vi "Zeile faerben.vi"(8 "error in (no error)":errorcluster caption="Fehler (Eingang, kein Fehler)", 9 "Offset für Start":i32, 10 "Anzahl":i32, 11 "Table (Eingang)":refnum<vi>) -> (0 "error out":errorcluster caption="Fehler (Ausgang)")   [LabVIEW 2020, in "FT-IR.lvlib" / "Spanfaktor.lvlib"]
uses:
  Spanfaktor.lvlib
  <vilib>/Utility/miscctls.llb/LVRowAndColumnTypeDef.ctl
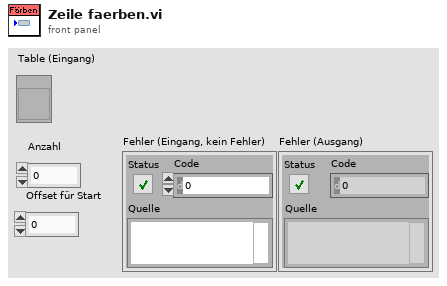
[diagram p1: front panel]
types:
  T1 = typedef "LVRowAndColumnTypeDef.ctl" = cluster{"Row":i32, "Column":i32}
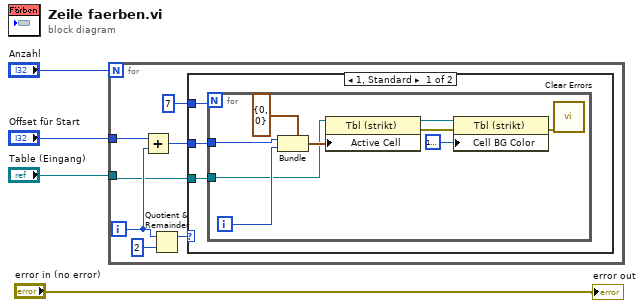
[diagram p0: block diagram]
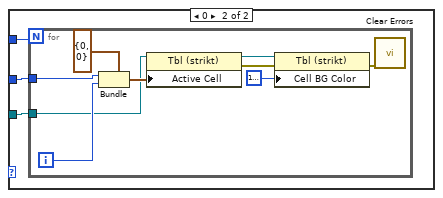
[diagram p2: hidden frame]
diagram:
  n1 = for {
    N: "Anzahl" -> [_]
    tunnel: "Table (Eingang)" -> [w8]
    tunnel: "Offset für Start" -> [w5]
    i -> [w9]
    n2 = Add(x=w5, y=w9) -> (x+y=w6:i32)
    n3 = Quotient & Remainder(x=w9, y=2) -> (x-y*floor(x/y)=w10:i32)  [unwired: 1 out]
    n4 = case shown="1, Standard" w10 {
      tunnel: w8 -> [w14 w26]
      tunnel: w6 -> [w13 w25]
      tunnel: 7 -> [w12 w24]
      frame 1, Default {
        n5 = for {
          N: w12 -> [_]
          tunnel: w14 -> [w18]
          tunnel: w13 -> [w20]
          i -> [w19]
          n6 = Bundle(cluster=T1 {"Row"=0, "Column"=0} ("Aktive Zelle:Aktive Zelle"), "Row"=w20, "Column"=w19) -> (w21:T1)
          n7 = property class="Tbl (strikt)"(reference=w18, "Active Cell"=w21) -> (reference out=w17:refnum<vi>, error out=w15:errorcluster)  [unwired: 1 in]
          n8 = property class="Tbl (strikt)"(reference=w17, error in=w15, "Cell BG Color"=u32 16777225) -> (error out=w16:errorcluster)  [unwired: 1 out]
          n9 = call <vilib>:"Clear Errors.vi"("error in (no error)"=w16) -> ()  [unwired: 5 in, 2 out]
        }
      }
      frame 0 {
        n10 = for {
          N: w24 -> [_]
          tunnel: w26 -> [w30]
          tunnel: w25 -> [w32]
          i -> [w31]
          n11 = Bundle(cluster=T1 {"Row"=0, "Column"=0} ("Aktive Zelle:Aktive Zelle"), "Row"=w32, "Column"=w31) -> (w33:T1)
          n12 = property class="Tbl (strikt)"(reference=w30, "Active Cell"=w33) -> (reference out=w29:refnum<vi>, error out=w27:errorcluster)  [unwired: 1 in]
          n13 = property class="Tbl (strikt)"(reference=w29, error in=w27, "Cell BG Color"=u32 16777238) -> (error out=w28:errorcluster)  [unwired: 1 out]
          n14 = call <vilib>:"Clear Errors.vi"("error in (no error)"=w28) -> ()  [unwired: 5 in, 2 out]
        }
      }
    }
  }
  "error out" <- "error in (no error)"
